vi "simulate arduino sensirion read with retry (sub-vi).vi"(7 "dirty data? (F)":bool, 8 "error in (no error)":errorcluster, 9 "expected num sensors (12)":i32=12, 10 "read byte count (512)":u32=512, 11 "VISA resource name":refnum<visa-resource-name>) -> (0 "error out":errorcluster, 1 "relative timestamp":dbl, 2 "sensor data array":T1[](array[typedef]) {"temperature" scale=293.15..303.15 scale format="%#_3g"}, 3 "VISA resource name out":refnum<visa-resource-name>, 4 "retry count":i32)   [LabVIEW 2021]
uses:
  controls/sensirion_flow_sensor_data.ctl
  type-defs/ardruino_sensirion_read_states.ctl
  type-defs/project_custom_error_codes_ring (type def).ctl
  <vilib>/numeric/Random Number (Range) DBL.vi
  <vilib>/ErrorRing/Error Ring.xnode
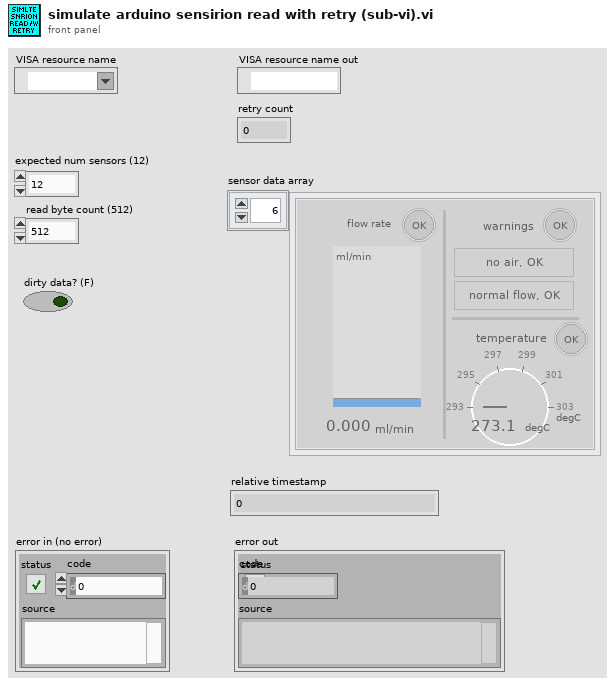
[diagram p1: front panel]
types:
  T1 = typedef "sensirion_flow_sensor_data.ctl" = cluster{"flow rate \n":dbl[unit], "flow val. status":bool, "temperature":dbl[unit], "temp. val status":bool, "air in line?":bool, "high flow?":bool, "flag. val status":bool}
  T2 = typedef "ardruino_sensirion_read_states.ctl" = enum16{"Initialize", "Read Buffer", "Retry", "Exit (Success)", "Fail", "Idle"}
  T3 = typedef "project_custom_error_codes_ring (type def).ctl" = i32
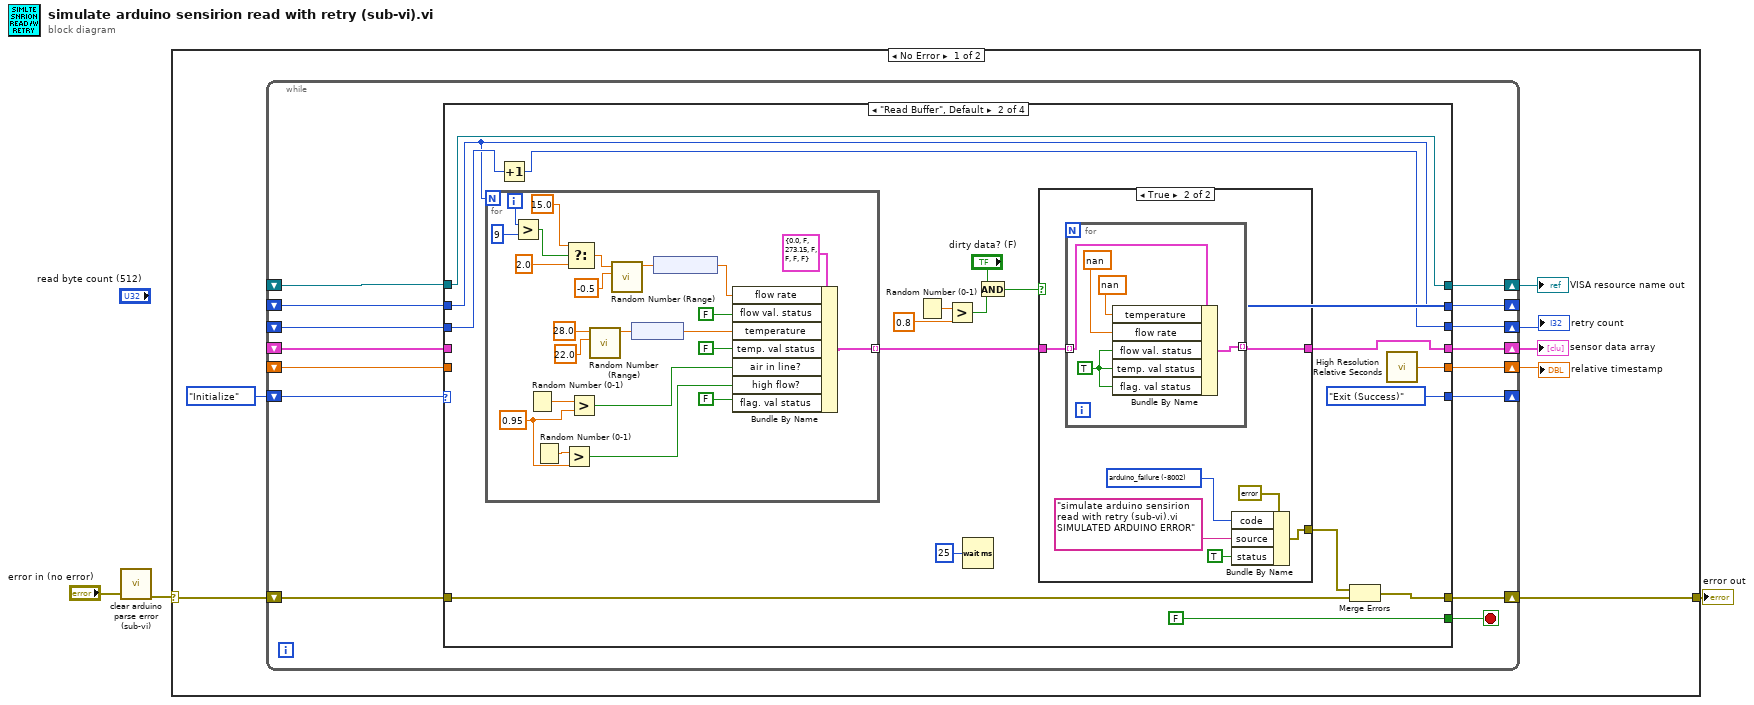
[diagram p0: block diagram]
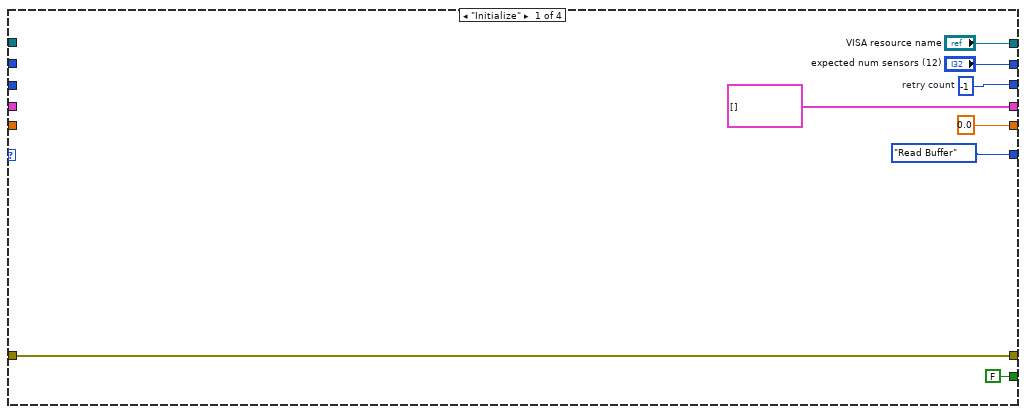
[diagram p2: hidden frame]
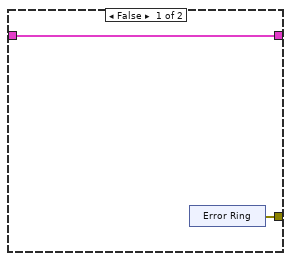
[diagram p3: hidden frame]
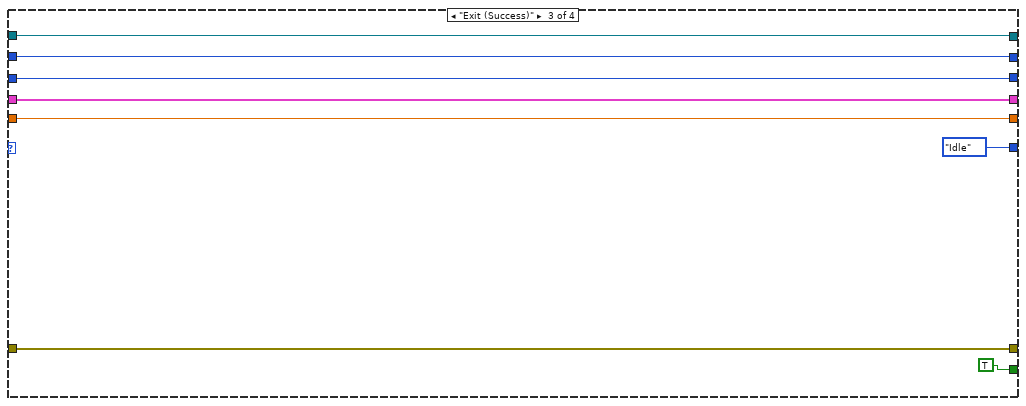
[diagram p4: hidden frame]
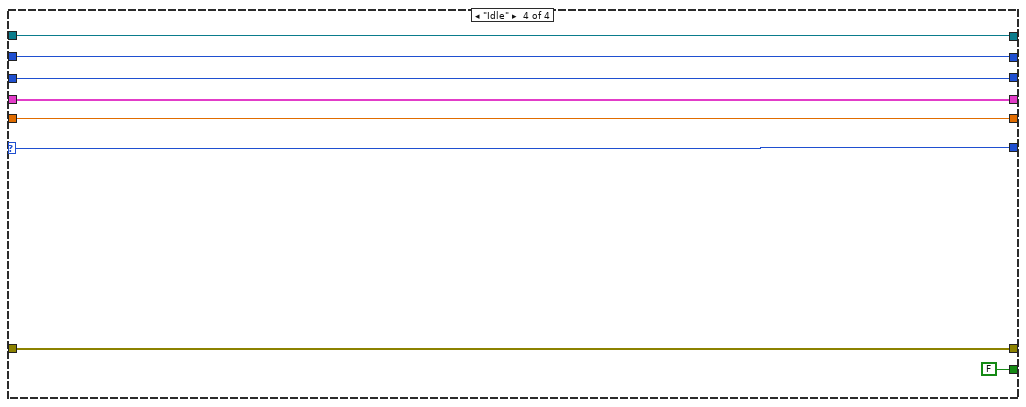
[diagram p5: hidden frame]
diagram:
  n1 = call "clear arduino parse error (sub-vi).vi"("error in"="error in (no error)") -> ("error out"=w1:errorcluster)  [unwired: 10 in]
  n2 = case shown="No Error" w1 {
    selector: w1 -> [w10 w106]
    tunnel: [w9 w106] -> w3
    frame No Error {
      n3 = while {
        shift-right: [w24] -> w9
        shift-left: w10 -> [w25]
        shift-right: [w23] -> w8
        shift-left: _ -> [w22]
        shift-right: [w21] -> _
        shift-left: _ -> [w20]
        shift-right: [w19] -> w5
        shift-left: _ -> [w18]
        shift-right: [w17] -> w7
        shift-left: _ -> [w16]
        shift-right: [w13] -> _
        shift-left: ardruino_sensirion_read_states."Initialize" ("Enum") -> [w14]
        shift-right: [w12] -> w4
        shift-left: _ -> [w11]
        stop <- w15 stop-if-true
        n4 = case shown="\"Read Buffer\", Default" w14 {
          selector: w14 -> [_ _ _ w101]
          tunnel: w25 -> [w28 w45 w92 w100]
          tunnel: ["VISA resource name" w46 w95 w105] -> w23
          tunnel: [w28 w36 w92 w100] -> w24
          tunnel: w22 -> [_ w46 w95 w105]
          tunnel: ["expected num sensors (12)" w44 w94 w104] -> w21
          tunnel: w20 -> [_ w44 w94 w104]
          tunnel: [w31 w50 w93 w103] -> w19
          tunnel: w18 -> [_ w49 w93 w103]
          tunnel: [T1[] [] ("sensor data array") w34 w97 w102] -> w17
          tunnel: w16 -> [_ _ w97 w102]
          tunnel: [FALSE FALSE TRUE FALSE] -> w15
          tunnel: [ardruino_sensirion_read_states."Read Buffer" ("Enum") ardruino_sensirion_read_states."Exit (Success)" ("Enum") ardruino_sensirion_read_states."Idle" ("Enum") w101] -> w13
          tunnel: [0.0 ("relative seconds") w47 w90 w98] -> w12
          tunnel: w11 -> [_ _ w90 w98]
          frame "Initialize" {
            w31 = -1  # retry count
          }
          frame "Read Buffer", Default {
            n5 = for {
              N: w44 -> [_]
              tunnel: [w73] -> w37 mode=indexing
              i -> [w67]
              w70 = 0.95 ("y")
              n6 = Greater?(x=w67, y=9) -> (0:w77:bool)
              n7 = Random Number (0-1)() -> (number: 0 to 1=w72:dbl)
              n8 = Random Number (0-1)() -> (number: 0 to 1=w71:dbl)
              n9 = Greater?(x=w71, y=w70) -> (0:w69:bool)
              n10 = Select(t=15.0 ("upper bound (100)"), s=w77, f=2.0) -> (s? t:f=w75:dbl)
              n11 = Greater?(x=w72, y=w70) -> (0:w68:bool)
              n12 = call-poly <vilib>:"Random Number (Range).vi"("lower bound (0)"=22.0, "upper bound (100)"=28.0) -> ("number"=w83:dbl)  [unwired: 9 in]
              n13 = call-poly <vilib>:"Random Number (Range).vi"("lower bound (0)"=-0.5, "upper bound (100)"=w75) -> ("number"=w80:dbl)  [unwired: 9 in]
              n14 = node(w83) -> (w82:dbl[unit])
              n15 = node(w80) -> (w79:dbl[unit])
              n16 = Bundle By Name(cluster=T1 {"flow rate \n"=0.0, "flow val. status"=FALSE, "temperature"=273.15, "temp. val status"=FALSE, "air in line?"=FALSE, "high flow?"=FALSE, "flag. val status"=FALSE} ("sensirion flow sensor data cluster"), "flow rate"=w79, "flow val. status"=FALSE, "temperature"=w82, "temp. val status"=FALSE, "air in line?"=w68, "high flow?"=w69, "flag. val status"=FALSE) -> (w73:T1)
            }
            n17 = Increment(x=w49) -> (x+1=w50:i32)
            n18 = Random Number (0-1)() -> (number: 0 to 1=w41:dbl)
            n19 = Greater?(x=w41, y=0.8) -> (0:w39:bool)
            n20 = Wait (ms)(milliseconds to wait=u32 25) -> ()  [unwired: 1 out]
            n21 = And(x="dirty data? (F)", y=w39) -> (x .and. y?=w38:bool)
            n22 = case shown="True" w38 {
              tunnel: w37 -> [w53 w61]
              tunnel: [w53 w60] -> w34
              tunnel: [w52 w56] -> w35
              frame False {
                n23 = xnode "Error Ring"() -> ("error out"=w52:errorcluster)
              }
              frame True {
                w57 = T3 -8002 items=["parse_failure"=-8001, "arduino_failure"=-8002] ("Ring")
                n24 = for {
                  tunnel: w61 -> [w66] mode=indexing
                  tunnel: [w64] -> w60 mode=indexing
                  w65 = TRUE ("flow val. status")
                  n25 = Bundle By Name(cluster=w66, "temperature"=dbl[unit] nan ("flow rate"), "flow rate"=dbl[unit] nan, "flow val. status"=w65, "temp. val status"=w65, "flag. val status"=w65) -> (w64:T1)
                }
                n26 = Bundle By Name(cluster=errorcluster {"status"=FALSE, "code"=0, "source"=""} ("error constant"), "code"=w57, "source"="simulate arduino sensirion read with retry (sub-vi).vi SIMULATED ARDUINO ERROR", "status"=TRUE) -> (w56:errorcluster)
              }
            }
            n27 = Merge Errors(w35, w45) -> (w36:errorcluster)
            n28 = call <vilib>:"High Resolution Relative Seconds.vi"() -> ("relative seconds"=w47:dbl)
          }
          frame "Exit (Success)" {
          }
          frame "Idle" {
          }
        }
      }
      "VISA resource name out" <- w8
      "sensor data array" <- w7
      "retry count" <- w5
      "relative timestamp" <- w4
    }
    frame Error {
    }
  }
  "error out" <- w3
